vi "Get Class VIs.vi"(8 "error in (no error)":errorcluster, 11 "class ref":refnum<vi>) -> (0 "error out":errorcluster, 3 "vi refs":refnum<vi>[](array[refnum]))   [LabVIEW 2017, in "Build Automation.lvlib"]
uses:
  Build Automation.lvlib
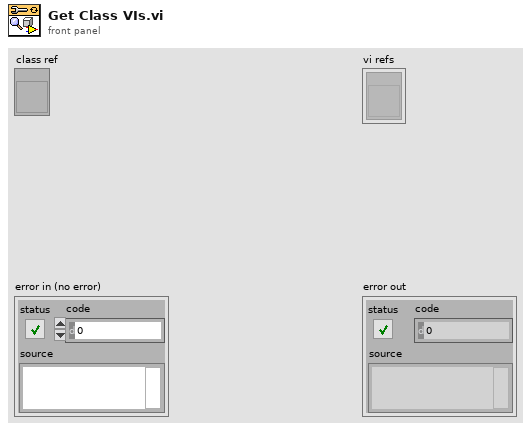
[diagram p1: front panel]
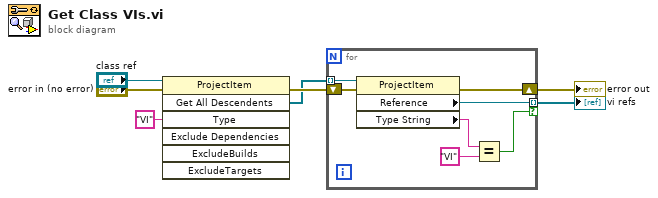
[diagram p0: block diagram]
diagram:
  n1 = invoke class="ProjectItem" method="Get All Descendents"(reference="class ref", error in="error in (no error)", "Type"="VI") -> (error out=w6:errorcluster, "All Descendents"=w5:refnum<vi>[])  [unwired: 4 in, 5 out]
  n2 = for {
    tunnel: w5 -> [w14] mode=indexing
    shift-right: [w11] -> w3
    shift-left: w6 -> [w12]
    tunnel: [w9] -> w2 mode=indexing if=w8
    n3 = property class="ProjectItem"(reference=w14, error in=w12) -> (error out=w11:errorcluster, "Reference"=w9:refnum<vi>, "Type String"=w10:string)  [unwired: 1 out]
    n4 = Equal?(x=w10, y="VI") -> (x = y?=w8:bool)
  }
  "error out" <- w3
  "vi refs" <- w2
